vi "Help.About.vi"(10 "Release Notes":string, 11 "SW Version":T1={"AppName"="Automated Test Station", "Company"="Kwest Engineering", "Version"="v1.0.1", "Description"="1/25/2016", "PN"=""}) -> ()   [LabVIEW 2024, in "EQMF.lvlib" / "Menu Utils.lvlib"]
uses:
  Menu Utils.lvlib
  Module/Module.SW Version Info.ctl
  Module/Module Utils.lvlib
panel:
  in  "Close":bool
  in  "Tab Control":enum32{"Version", "Release Notes"}(tab)
  out "PN":string
  out "Name":string
  out "By":string
  out "Version":string
  out "Description":string
  out "Labview Runtime Engine":string
  out "Release Notes 2":string
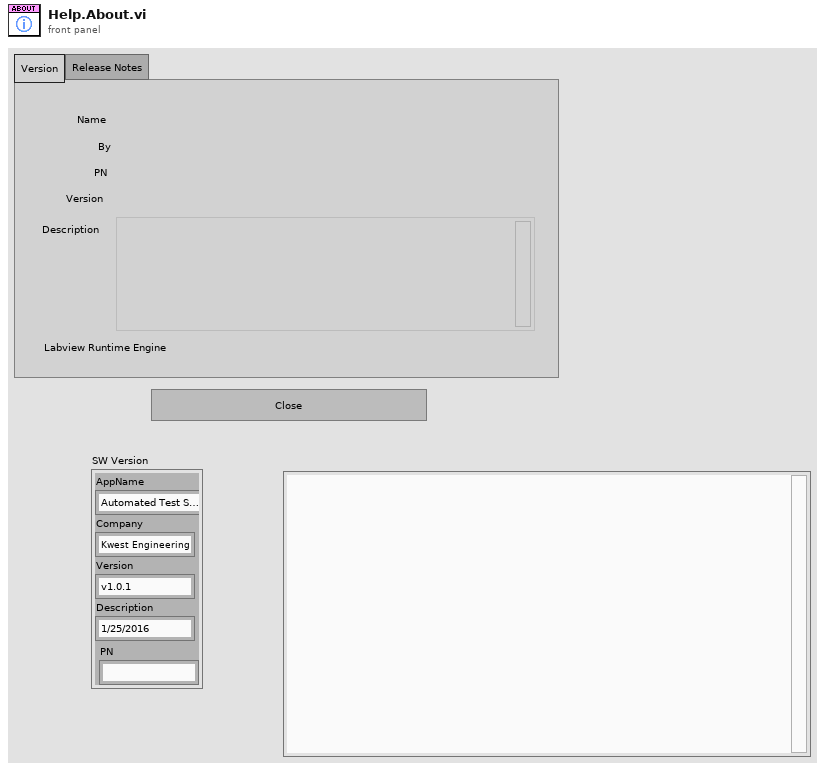
[diagram p1: front panel]
types:
  T1 = typedef "EQMF.lvlib/Module Utils.lvlib/Module.SW Version Info.ctl" = cluster{"AppName":string, "Company":string, "Version":string, "Description":string, "PN":string}
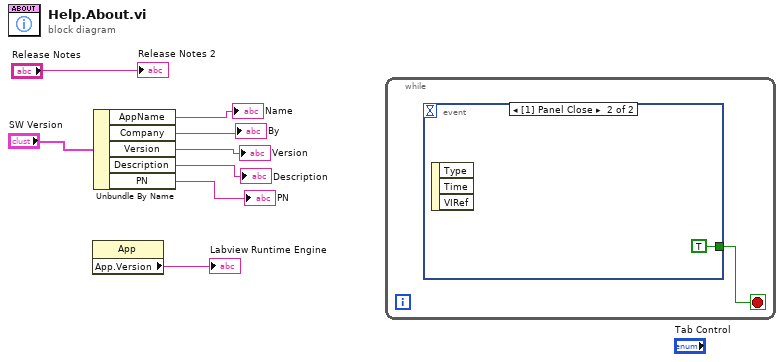
[diagram p0: block diagram]
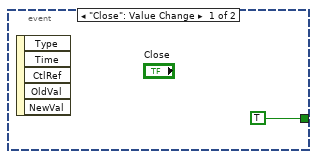
[diagram p2: hidden frame]
diagram:
  n1 = property class="App"() -> ("App.Version"=→"Labview Runtime Engine":string)  [unwired: 2 in, 2 out]
  n2 = Unbundle By Name("SW Version") -> ("AppName"=→"Name":string, "Company"=→"By":string, "Version"=→"Version":string, "Description"=→"Description":string, "PN"=→"PN":string)
  n3 = while {
    stop <- w9 stop-if-true
    n4 = event shown="[1] Panel Close" {
      selector: _ -> [_ _]
      dyn-events: _ -> [_ _]
      timeout: _ -> [_ _]
      tunnel: [TRUE TRUE] -> w9
      event "Close": Value Change {
        n5 = event-data() -> ()  [unwired: 1 in, 5 out]
      }
      event Panel Close {
        n6 = event-data() -> ()  [unwired: 1 in, 3 out]
      }
    }
  }
  "Release Notes 2" <- "Release Notes"
